vi "Set_cursor_position.vi"() -> ()   [LabVIEW 2010]
panel:
  in  "Field_Astrom":T1 {"CRVAL" format="%.6g"; "CD" format="%_7g"}
  in  "table Y":dbl
  in  "table X":dbl
  out "cursor DEC":dbl
  out "cursor RA":dbl
  out "table Y":dbl
  out "table X":dbl
  in  "DEC tel":dbl
  in  "RA tel":dbl
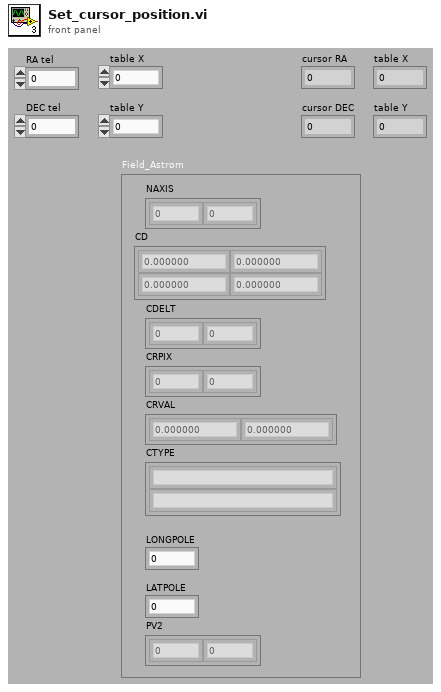
[diagram p1: front panel]
types:
  T1 = cluster{"NAXIS":dbl[], "CD":dbl[][], "CDELT":dbl[], "CRPIX":dbl[], "CTYPE":string[], "CRVAL":dbl[], "LONGPOLE":dbl, "LATPOLE":dbl, "PV2":dbl[]}
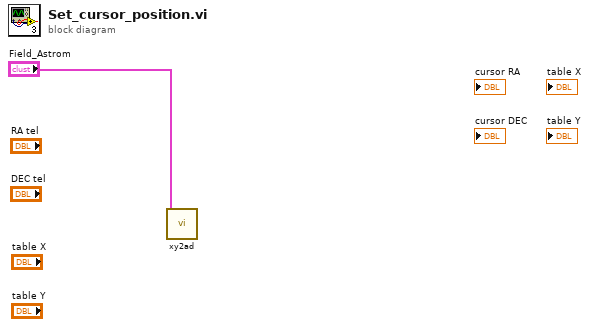
[diagram p0: block diagram]
diagram:
  n1 = call "xy2ad.vi"("Astrometry"="Field_Astrom") -> ()  [unwired: 8 in, 3 out]
